vi "DMM Already Connected.vi"(2 "error in (no error)":errorcluster, 3 "Control Set Array":T1[](array[typedef]), 4 "Index":i32, 5 "DMM Address":refnum<visa-resource-name>="GPIB0::5::INSTR") -> (0 "error out":errorcluster, 1 "Conflict Exists":bool)   [LabVIEW 2020]
uses:
  Typedefs/DMM Control Variable References.ctl
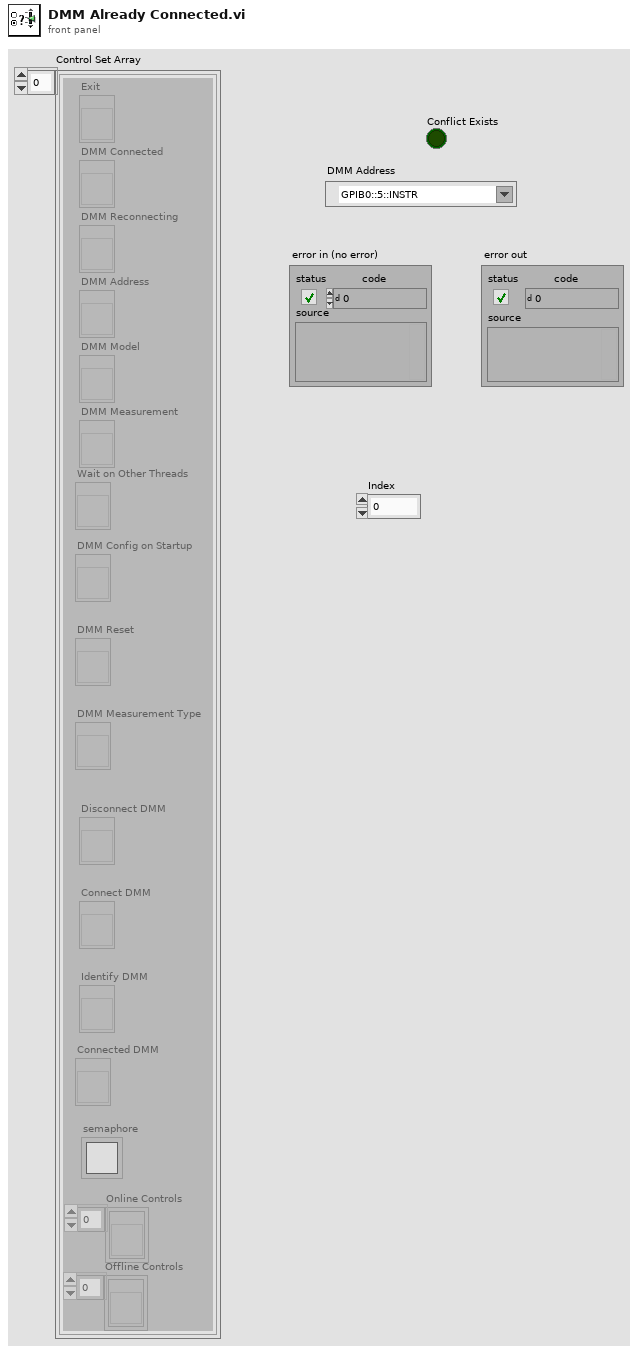
[diagram p1: front panel]
types:
  T1 = typedef "DMM Control Variable References.ctl" = cluster{"Exit":refnum<vi>, "DMM Connected":refnum<vi>, "DMM Reconnecting":refnum<vi>, "DMM Address":refnum<vi>, "DMM Model":refnum<vi>, "DMM Measurement":refnum<vi>, "Wait on Other Threads":refnum<vi>, "DMM Reset":refnum<vi>, "DMM Config on Startup":refnum<vi>, "DMM Measurement Type":refnum<vi>, "Disconnect DMM":refnum<vi>, "Connect DMM":refnum<vi>, "Identify DMM":refnum<vi>, "Connected DMM":refnum<vi>, "semaphore":T2, "Online Controls":refnum<vi>[], "Offline Controls":refnum<vi>[]}
  T2 = typedef "Semaphore RefNum" = refnum<k1>
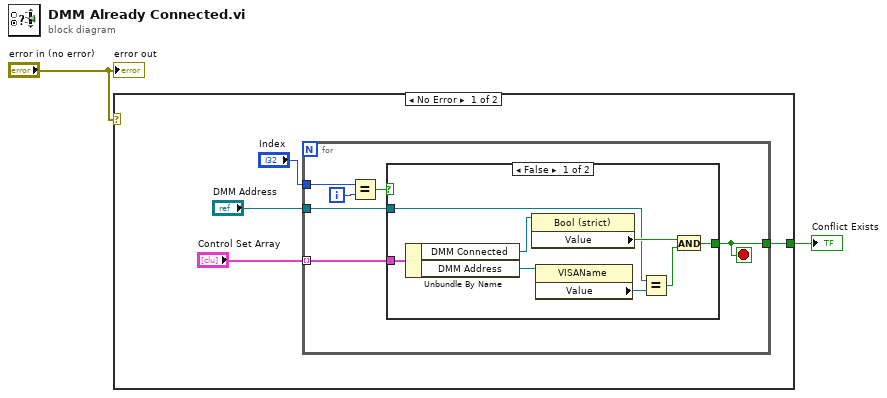
[diagram p0: block diagram]
diagram:
  n1 = case shown="No Error" "error in (no error)" {
    tunnel: [w3 _] -> w1
    frame No Error {
      n2 = for {
        tunnel: "Control Set Array" -> [w12] mode=indexing
        tunnel: "DMM Address" -> [w11]
        tunnel: "Index" -> [w9]
        tunnel: [w7] -> w3
        i -> [w10]
        stop <- w7 stop-if-true
        n3 = Equal?(x=w9, y=w10) -> (x = y?=w8:bool)
        n4 = case shown="False" w8 {
          tunnel: w12 -> [w20 _]
          tunnel: w11 -> [w15 _]
          tunnel: [w13 _] -> w7
          frame False {
            n5 = Unbundle By Name(w20) -> ("DMM Connected"=w19:refnum<vi>, "DMM Address"=w18:refnum<vi>)
            n6 = property class="Bool (strict)"(reference=w19) -> ("Value"=w17:bool)  [unwired: 1 in, 2 out]
            n7 = property class="VISAName"(reference=w18) -> ("Value"=w16:refnum<visa-resource-name>)  [unwired: 1 in, 2 out]
            n8 = Equal?(x=w15, y=w16) -> (x = y?=w14:bool)
            n9 = And(x=w17, y=w14) -> (x .and. y?=w13:bool)
          }
          frame True {
          }
        }
      }
    }
    frame Error {
    }
  }
  "Conflict Exists" <- w1
  "error out" <- "error in (no error)"
